vi "Configure Sequence Edge.vi"(0 "VISA resource name":refnum<visa-resource-name>, 5 "Trigger Source (0: Channel 1)":u16(ring) items=["Channel 1", "Channel 2", "Channel 3", "Channel 4", "DIG 0", "DIG 1", "DIG 2", "DIG 3", "DIG 4", "DIG 5", "DIG 6", "DIG 7", "DIG 8", "DIG 9", "DIG 10", "DIG 11", "DIG 12", "DIG 13", "DIG 14", "DIG 15", "EXT"], 7 "Slope (1: Positive)":u16(ring)=1 items=["Negative", "Positive"], 9 "Edge (0: Edge 1)":u16(ring) items=["Edge 1", "Edge 2"], 11 "error in (no error)":errorcluster) -> (4 "VISA resource name out":refnum<visa-resource-name>, 15 "error out":errorcluster)   [LabVIEW 2017, in "Agilent 6000 Series.lvlib"]
doc: "This VI configures the Sequence trigger. You specify the edge, source and slope with the Edge, Trigger Source and Slope parameters.\n\n<B>NOTE:</B>\n\nThis VI is only valid for 6000 Series models. An error will be thrown if this VI is run with 5000 Series scopes."
uses:
  <instrlib>/Agilent 6000 Series/Agilent 6000 Series.lvlib
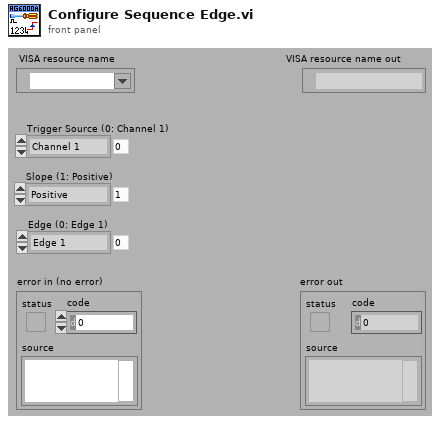
[diagram p1: front panel]
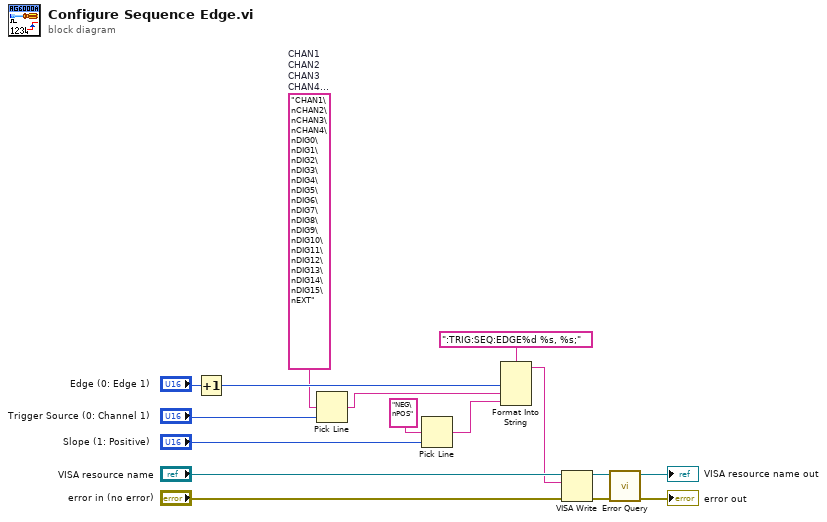
[diagram p0: block diagram]
diagram:
  w6 = "CHAN1\nCHAN2\nCHAN3\nCHAN4\nDIG0\nDIG1\nDIG2\nDIG3\nDIG4\nDIG5\nDIG6\nDIG7\nDIG8\nDIG9\nDIG10\nDIG11\nDIG12\nDIG13\nDIG14\nDIG15\nEXT"  # CHAN1 CHAN2 CHAN3 CHAN4 DIG0 DIG1 DIG2 DIG3 DIG4 DIG5 DIG6 DIG7 DIG8 DIG9 DIG10 DIG11 DIG12 DIG13 DIG14 DIG15 EXT
  n1 = Increment(x="Edge (0: Edge 1)") -> (x+1=w8:u16)
  n2 = Pick Line(multi-line string=w6, line index="Trigger Source (0: Channel 1)") -> (output string=w4:string)  [unwired: 1 in]
  n3 = Pick Line(multi-line string="NEG\nPOS", line index="Slope (1: Positive)") -> (output string=w1:string)  [unwired: 1 in]
  n4 = Format Into String(format string=":TRIG:SEQ:EDGE%d %s, %s;" ("Source Command"), w8, w4, w1) -> (resulting string=w9:string)  [unwired: 2 in, 1 out]
  n5 = VISA Write(VISA resource name="VISA resource name", write buffer=w9, error in (no error)="error in (no error)") -> (VISA resource name out=w12:refnum<visa-resource-name>, error out=w11:errorcluster)  [unwired: 1 out]
  n6 = call <instrlib>:"Error Query.vi"("error in (no error)"=w11, "VISA resource name"=w12) -> ("error out"=→"error out":errorcluster, "VISA resource name out"=→"VISA resource name out":refnum<visa-resource-name>)  [unwired: 6 in, 2 out]
